vi "LVClass_Image get image general information.vi"(0 "Image in":refnum<class "Image.lvclass">, 11 "error in (no error)":errorcluster) -> (4 "Image out":refnum<class "Image.lvclass">, 6 "Acquisition information":T1, 15 "error out":errorcluster)   [LabVIEW 2020, in "Image.lvclass"]
doc: "Get metadata from Image object.\n\n--------------------------------------------------------------------------------\n\n<B>ImageIn </B> : Image object.\n<B>ImageOut </B> : Image object.\n<B>haso_serial_number </B> : Haso serial number.\n<B>camera_serial_number </B> : Camera serial number.\n<B>exposure_time_applied </B> : Exposure duration applied (us).\n<B>exposure_time_requested </B> : Exposure duration requested (us).\n<B>gain </B> : Applied gain (SI).\n<B>nb_summed_images </B> : Number of summed images.\n<B>is_smearing_removed </B> : Smearing_removed.\n<B>is_background_removed </B> : Background_removed.\n<B>trigger_type </B> : Trigger mode.\n<B>time_stamp </B> : Date of the acquired Image.\n<B>max_level </B> : Max level value.\n<B>comments </B> : Comments.\n<B>ErrorIn </B> : Error\n<B>ErrorOut </B> : Error\n\n--------------------------------------------------------------------------------"
uses:
  Image.lvclass
  Controls/Image general information.ctl
  Image.lvclass/Image.ctl
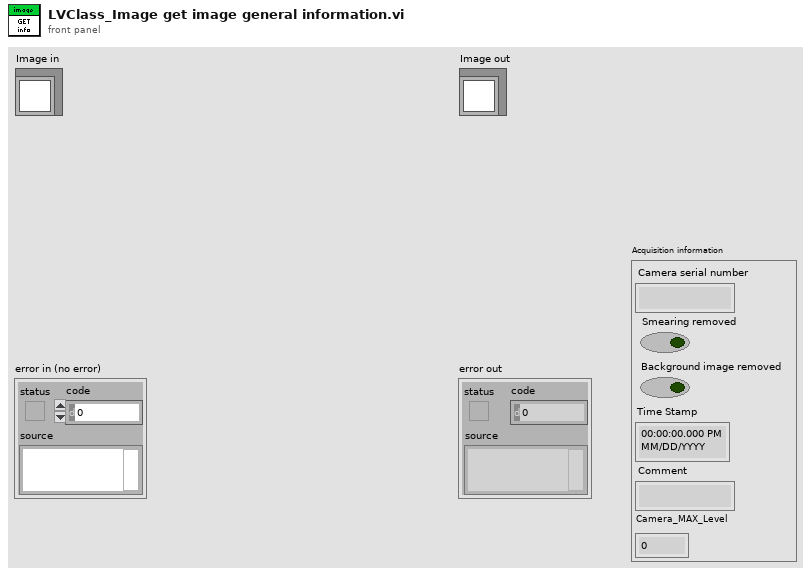
[diagram p1: front panel]
types:
  T1 = typedef "Image general information.ctl" = cluster{"Camera serial number":string, "Smearing removed":bool, "Background image removed":bool, "Time Stamp":timestamp, "Comment":string, "Camera_MAX_Level":i32}
  T2 = typedef "ClassID.ctl" = i64
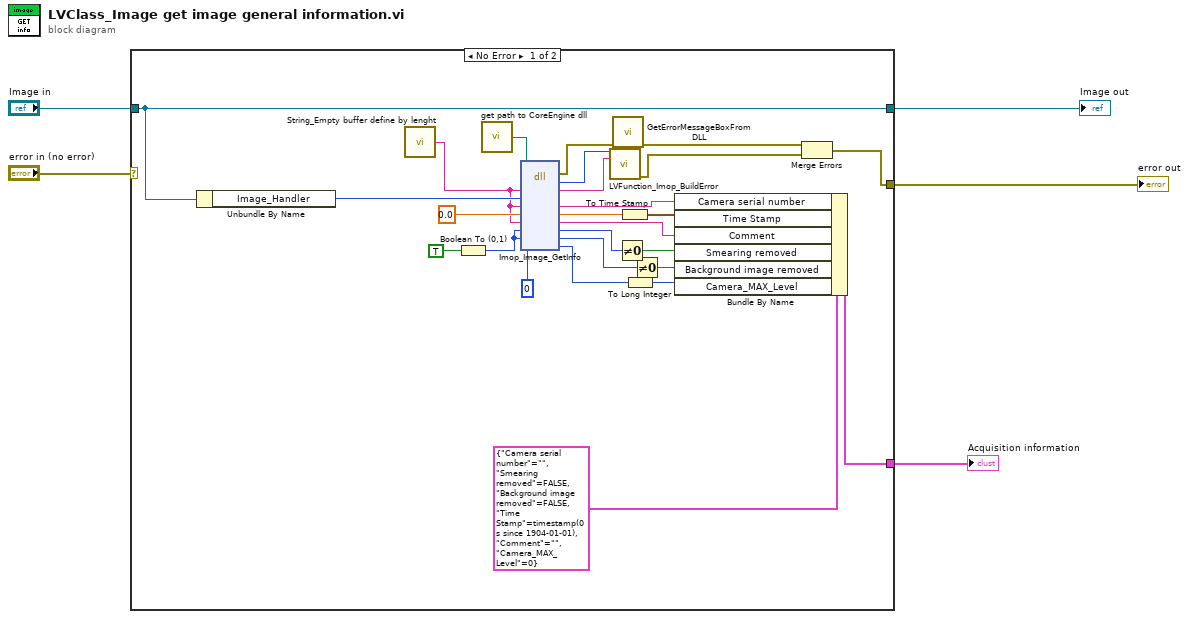
[diagram p0: block diagram]
diagram:
  n1 = case shown="No Error" "error in (no error)" {
    selector: "error in (no error)" -> [_ w33]
    tunnel: [w12 w33] -> w4
    tunnel: [w9 w32] -> w2
    tunnel: "Image in" -> [w9 w32]
    tunnel: [w26 _] -> w1
    frame No Error {
      n2 = Unbundle By Name(w9) -> ("Image_Handler"=w31:T2)
      n3 = call "String_Empty buffer define by lenght.vi"() -> ("Empty buffer"=w10:string)  [unwired: 1 in]
      n4 = Boolean To (0,1)(Boolean=TRUE) -> (0, 1=w19:i16)
      n5 = call "get path to CoreEngine dll.vi"() -> ("path to wavekit library"=w28:path)  [unwired: 14 in, 1 out]
      n6 = dll-call lib="D:/2_trunk/Soft_haso/ImOpCoreEngine4_LV2011/DLLs/ImopEngine4_vc100.dll" fn="Imop_Image_GetInfo"(path in=w28, "message"=w10, "Image compat"=w31, "camera_serial_number"=w10, "time_stamp"=0.0, "comments"=w10, "smearing_removed"=w19, "background_removed"=w19, "max_level"=i64 0) -> (error out=w27:errorcluster, "return type"=w30:i32, "message"=w29:string, "camera_serial_number"=w11:string, "time_stamp"=w25:dbl, "comments"=w6:string, "smearing_removed"=w18:u8, "background_removed"=w17:u8, "max_level"=w22:i64)  [unwired: 3 in, 1 out]
      n7 = call "LVFunction_Imop_BuildError.vi"("code"=w30, "String to Prepend to source (\"\")"=w29) -> ("error out"=w13:errorcluster)  [unwired: 13 in]
      n8 = call "GetErrorMessageBoxFromDLL.vi"("error IN"=w27) -> ("error OUT"=w14:errorcluster)  [unwired: 10 in]
      n9 = Not Equal To 0?(x=w18) -> (x != 0?=w16:bool)
      n10 = To Time Stamp(1:w25) -> (0:w7:timestamp)
      n11 = To Long Integer(number=w22) -> (32bit integer=w21:i32)
      n12 = Not Equal To 0?(x=w17) -> (x != 0?=w15:bool)
      n13 = Bundle By Name(cluster=T1 {"Camera serial number"="", "Smearing removed"=FALSE, "Background image removed"=FALSE, "Time Stamp"=timestamp(0 s since 1904-01-01), "Comment"="", "Camera_MAX_Level"=0} ("Acquisition information"), "Camera serial number"=w11, "Time Stamp"=w7, "Comment"=w6, "Smearing removed"=w16, "Background image removed"=w15, "Camera_MAX_Level"=w21) -> (w26:T1)
      n14 = Merge Errors(w14, w13) -> (w12:errorcluster)
    }
    frame Error {
    }
  }
  "error out" <- w4
  "Image out" <- w2
  "Acquisition information" <- w1
